vi "Prepare Scan Data to Array.vi"(8 "error in (no error)":errorcluster, 11 "Packet A in":refnum<class "Packet A.lvclass">) -> (0 "error out":errorcluster, 2 "Distance x Angule":cluster{"Magnitude":dbl, "Phase":dbl}[](array[cluster]), 3 "Packet A out":refnum<class "Packet A.lvclass">)   [LabVIEW 2019, in "Packet A.lvclass"]
uses:
  Packet A.lvclass
  Packet A.lvclass/Packet A.ctl
  Packet/Packet.lvclass
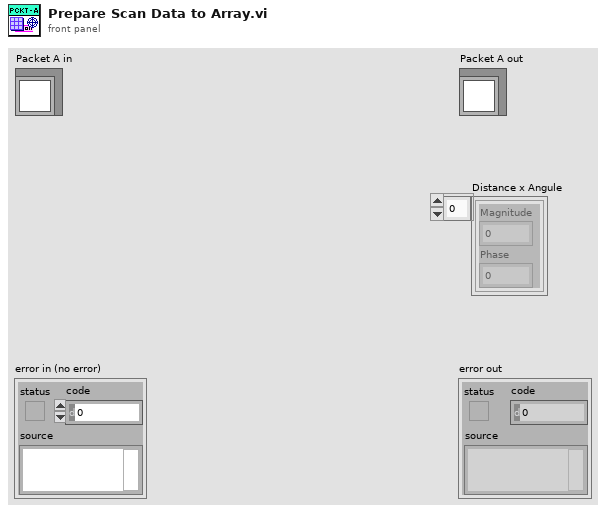
[diagram p1: front panel]
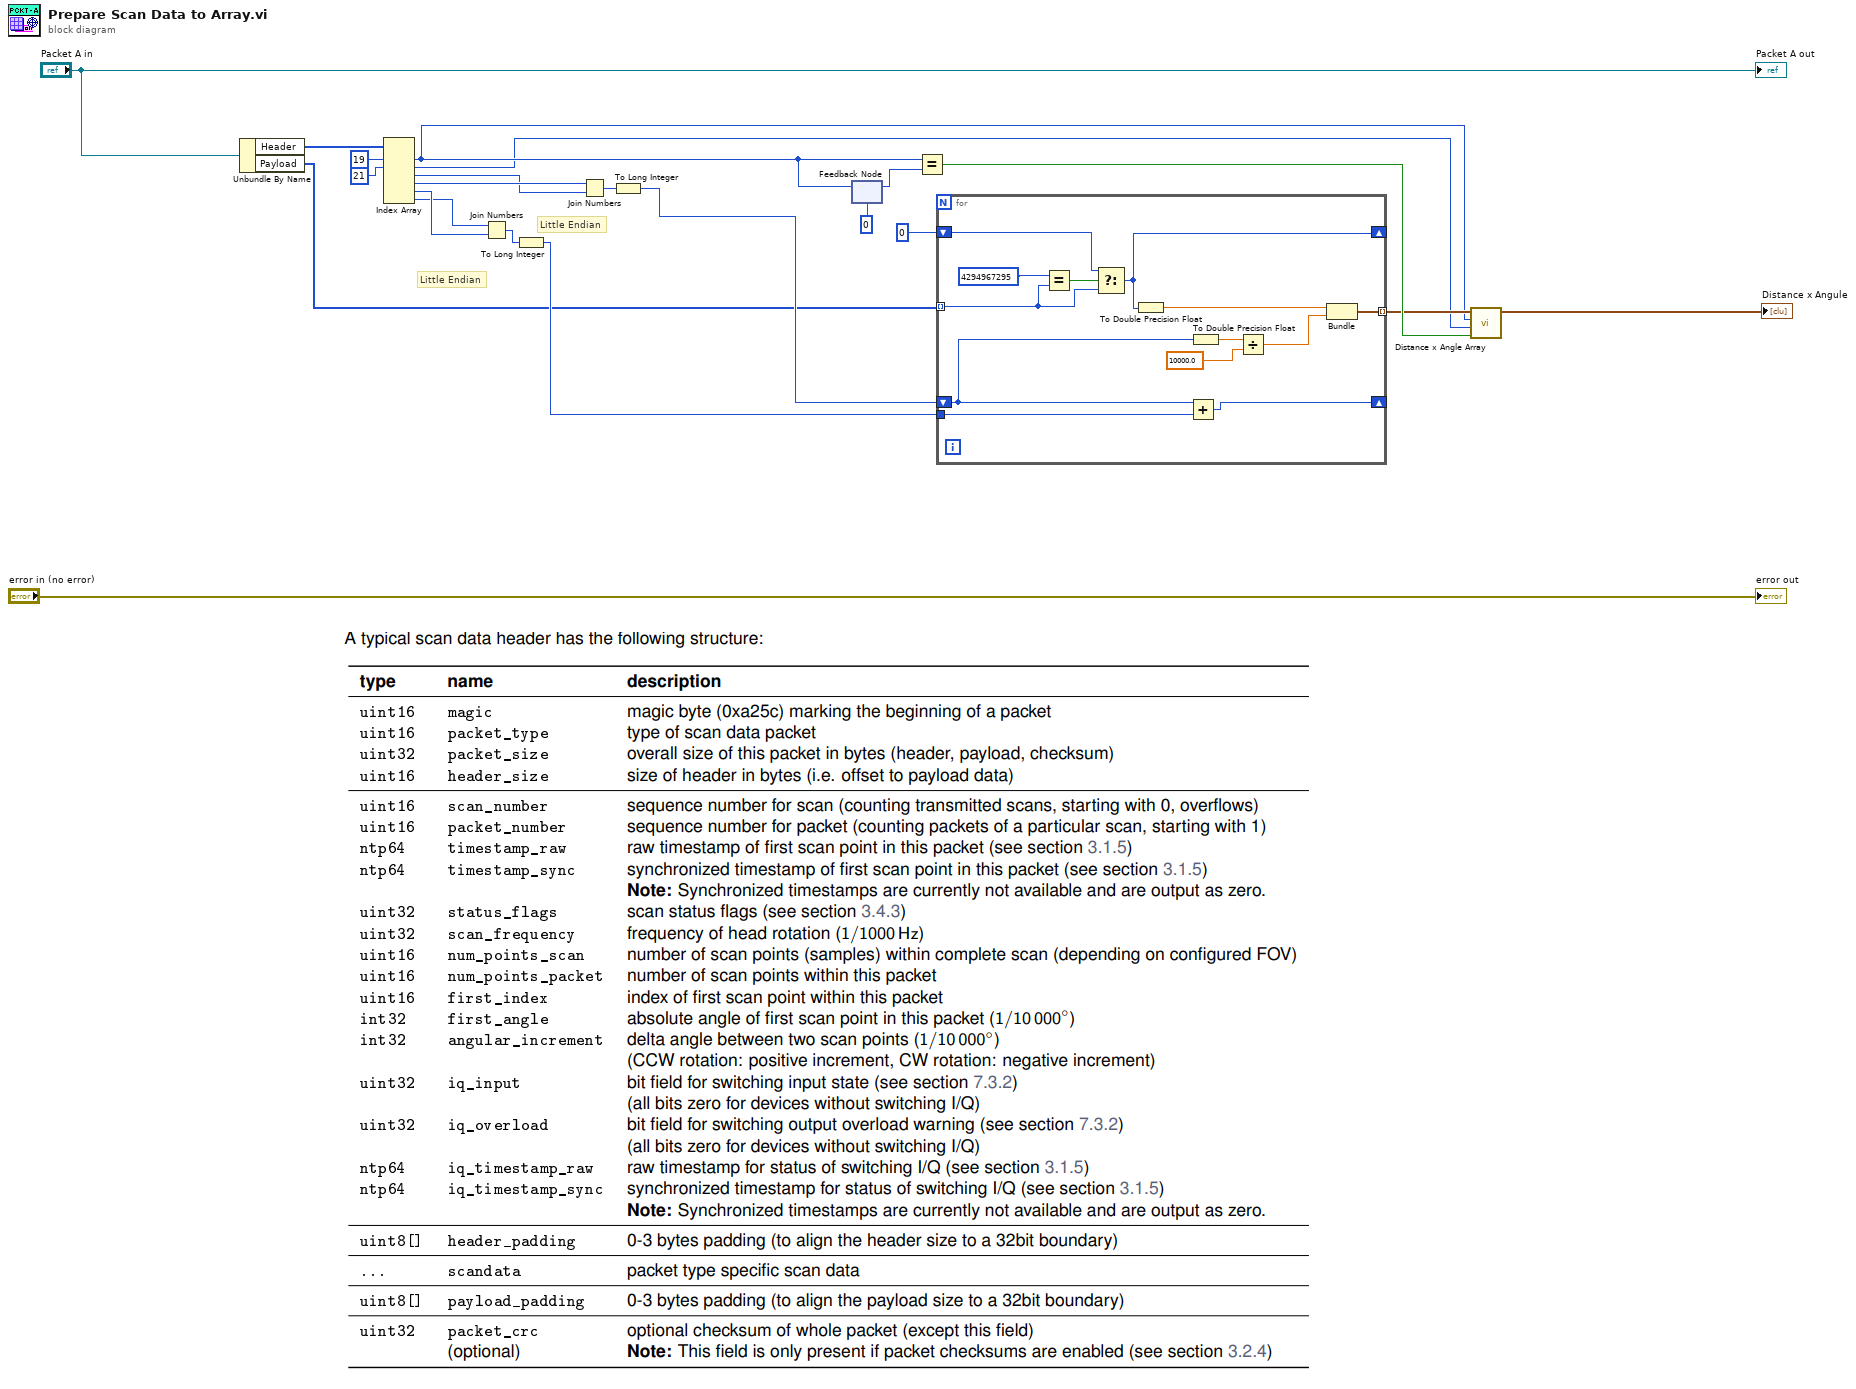
[diagram p0: block diagram]
diagram:
  # "Little Endian"
  # "Little Endian"
  n1 = Unbundle By Name("Packet A in") -> ("Header"=w10:u16[], "Payload"=w1:u32[])
  n2 = Index Array "Index Array"(array=w10, index #1=19 ("index"), index #2=21 ("index")) -> (element #1=w14:u16, element #2=w13:u16, element #3=w5:u16, element #4=w6:u16, element #5=w3:u16, element #6=w2:u16)  [unwired: 4 in]
  n3 = Join Numbers(hi=w2, lo=w3) -> ((hi.lo)=w4:u32)
  n4 = To Long Integer(number=w4) -> (32bit integer=w12:i32)
  n5 = Join Numbers(hi=w6, lo=w5) -> ((hi.lo)=w7:u32)
  n6 = To Long Integer(number=w7) -> (32bit integer=w11:i32)
  n7 = feedback #1(u16 0 ("Num_Points_Scan")) -> (w18:u16)
  n8 = feedback-in #1(w14) -> ()
  n9 = Equal?(x=w14, y=w18) -> (x = y?=w20:bool)
  n10 = for {
    tunnel: w1 -> [w24] mode=indexing
    tunnel: w12 -> [w35]
    shift-right: [w34] -> _
    shift-left: w11 -> [w32]
    tunnel: [w28] -> w19 mode=indexing
    shift-right: [w23] -> _
    shift-left: u32 0 -> [w25]
    n11 = Equal?(x=u32 4294967295, y=w24) -> (x = y?=w26:bool)
    n12 = Select(t=w25, s=w26, f=w24) -> (s? t:f=w23:u32)
    n13 = To Double Precision Float(number=w23) -> (double precision float=w30:dbl)
    n14 = Add(x=w32, y=w35) -> (x+y=w34:i32)
    n15 = To Double Precision Float(number=w32) -> (double precision float=w33:dbl)
    n16 = Divide(x=w33, y=10000.0) -> (x/y=w29:dbl)
    n17 = Bundle(w30, w29) -> (w28:cluster{dbl, dbl})  [unwired: 1 in]
  }
  n18 = call "Distance x Angle Array.vi"("Boolean"=w20, "First Index"=w13, "Num_Points_Scan"=w14, "Distance x Angle In"=w19) -> ("Distance x Angule"=→"Distance x Angule":cluster{"Magnitude":dbl, "Phase":dbl}[])  [unwired: 7 in]
  "error out" <- "error in (no error)"
  "Packet A out" <- "Packet A in"
